vi "Tree.vi"   [LabVIEW 2016, in "Control Experiment SM.lvclass"]
uses:
  Control Experiment SM/Control Experiment SM.lvclass
  <userlib>/LevyLab/Krohn Hite 7008/Instrument.KH7008.lvclass
  <userlib>/LevyLab/Lockin-Multichannel/Instrument.Lockin/Instrument.Lockin.lvclass
  Typedefs/Instrument--enum.ctl
types:
  T1 = typedef "Control Experiment SM.lvclass/Instrument--enum.ctl" = enum16{"----- AFM/EBL -----", "AGILENT", "CYPHER", "Gemini2", "JEOL", "MFP3D", "----- Cryostat -----", "CF900", "DR200", "MNK", "PPMS 1", "PPMS 2", "PPMS 3", "----- Optics -----", "THz 1", "THz 2"}
  T2 = typedef "Control Experiment SM.lvclass/Instruments--cluster.ctl" = cluster{"KH7008":refnum<class "Instrument.KH7008.lvclass">[], "Lockin":refnum<class "Instrument.Lockin.lvclass">, "Temperature":refnum<class "Instrument.Cryostat.lvclass">, "Magnet":refnum<class "Instrument.Cryostat.lvclass">, "Rotator":refnum<class "Instrument.Cryostat.lvclass">, "Level":refnum<class "Instrument.Cryostat.lvclass">, "Capacitance Bridge":refnum<class "Instrument.CBridge.lvclass">, "Optical Delay Line":refnum<class "Instrument.OpticalDelayLine.lvclass">, "Strain Cell":refnum<class "Instrument.Strain.lvclass">, "VNA":refnum<class "Instrument.VNA.lvclass">, "Voltage Source":refnum<class "Instrument.VSource.lvclass">}
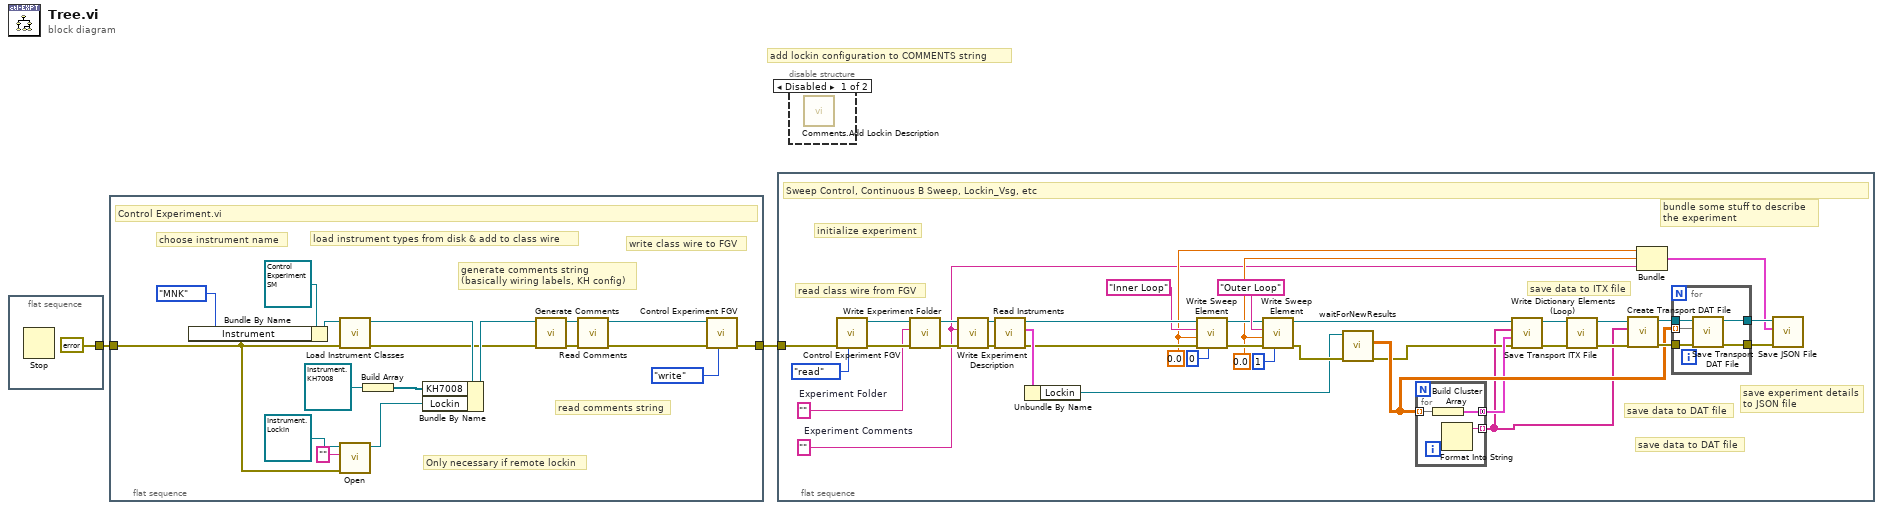
[diagram p0: block diagram]
diagram:
  # "add lockin configuration to COMMENTS string"
  n1 = flat-sequence {
    tunnel: [errorcluster {"status"=FALSE, "code"=0, "source"=""} ("error in (no error)")] -> w2
    frame #0 {
      n2 = Stop() -> ()  [unwired: 1 in]
    }
  }
  n3 = flat-sequence {
    tunnel: w2 -> [w10]
    tunnel: [w9] -> w1
    frame #0 {
      # "choose instrument name"
      # "Only necessary if remote lockin"
      # "write class wire to FGV"
      # "read comments string"
      # "generate comments string\n(basically wiring labels, KH config)"
      # "load instrument types from disk & add to class wire"
      # "Control Experiment.vi"
      n4 = Bundle By Name(cluster=refnum<class "Control Experiment SM.lvclass"> refnum ("Control Experiment.lvclass"), "Instrument"=Instrument--enum."MNK" ("Experiment.Instrument")) -> (w6:refnum<class "Control Experiment SM.lvclass">)
      n5 = call "Load Instrument Classes.vi"("error in (no error)"=w10, "Control Experiment.lvclass"=w6) -> ("error out"=w14:errorcluster, "Control Experiment out"=w16:refnum<class "Control Experiment SM.lvclass">)  [unwired: 8 in]
      n6 = call-dynamic "Open.vi"("error in (no error)"=w10, "Address"="", "Instrument.Lockin in"=refnum<class "Instrument.Lockin.lvclass"> refnum ("Instruments.Lockin")) -> ("Instrument.Lockin out"=w18:refnum<class "Instrument.Lockin.lvclass">)  [unwired: 7 in, 1 out]
      n7 = Build Array(refnum<class "Instrument.KH7008.lvclass"> refnum ("Instruments.KH7008")) -> (w4:refnum<class "Instrument.KH7008.lvclass">[])
      n8 = Bundle By Name(cluster=w16, "KH7008"=w4, "Lockin"=w18) -> (w15:refnum<class "Control Experiment SM.lvclass">)
      n9 = call "Generate Comments.vi"("error in (no error)"=w14, "Control Experiment"=w15) -> ("error out"=w21:errorcluster, "Control Experiment out"=w20:refnum<class "Control Experiment SM.lvclass">)  [unwired: 6 in, 1 out]
      n10 = call "Read Comments.vi"("error in (no error)"=w21, "Control Experiment in"=w20) -> ("error out"=w13:errorcluster, "Control Experiment out"=w12:refnum<class "Control Experiment SM.lvclass">)  [unwired: 7 in, 1 out]
      n11 = call "Control Experiment FGV.vi"("Function"=enum16{"read", "write"}."write", "error in (no error)"=w13, "Control Experiment.lvclass"=w12) -> ("error out"=w9:errorcluster)  [unwired: 7 in, 1 out]
    }
  }
  n12 = flat-sequence {
    tunnel: w1 -> [w58]
    frame #0 {
      w31 = ""  # Experiment Comments
      w30 = ""  # Experiment Folder
      w32 = 0.0
      w33 = 0.0
      # "initialize experiment"
      # "save experiment details\nto JSON file"
      # "save data to DAT file"
      # "save data to DAT file"
      # "save data to ITX file"
      # "bundle some stuff to describe\nthe experiment"
      # "read class wire from FGV"
      # "Sweep Control, Continuous B Sweep, Lockin_Vsg, etc"
      n13 = call "Control Experiment FGV.vi"("Function"=enum16{"read", "write"}."read", "error in (no error)"=w58) -> ("error out"=w54:errorcluster, "Control Experiment.lvclass out"=w53:refnum<class "Control Experiment SM.lvclass">)  [unwired: 8 in]
      n14 = call "Write Experiment Folder.vi"("error in (no error)"=w54, "Experiment Folder"=w30, "Control Experiment in"=w53) -> ("error out"=w55:errorcluster, "Control Experiment out"=w56:refnum<class "Control Experiment SM.lvclass">)  [unwired: 7 in]
      n15 = call "Write Experiment Description.vi"("error in (no error)"=w55, "Experiment Description"=w31, "Control Experiment in"=w56) -> ("error out"=w52:errorcluster, "Control Experiment out"=w51:refnum<class "Control Experiment SM.lvclass">)  [unwired: 7 in]
      n16 = call "Read Instruments.vi"("error in (no error)"=w52, "Control Experiment in"=w51) -> ("error out"=w49:errorcluster, "Instruments"=w50:T2, "Control Experiment out"=w48:refnum<class "Control Experiment SM.lvclass">)  [unwired: 7 in]
      n17 = Unbundle By Name(w50) -> ("Lockin"=w29:refnum<class "Instrument.Lockin.lvclass">)
      n18 = call "Write Sweep Element.vi"("loop index"=0, "error in (no error)"=w49, "value"=w33, "key"="Inner Loop", "Control Experiment in"=w48) -> ("error out"=w42:errorcluster, "Control Experiment out"=w43:refnum<class "Control Experiment SM.lvclass">)  [unwired: 5 in]
      n19 = call "Write Sweep Element.vi"("loop index"=1, "error in (no error)"=w42, "value"=w32, "key"="Outer Loop", "Control Experiment in"=w43) -> ("error out"=w41:errorcluster, "Control Experiment out"=w26:refnum<class "Control Experiment SM.lvclass">)  [unwired: 5 in]
      n20 = call <userlib>:"waitForNewResults.vi"("error in (no error)"=w41, "Instrument.Lockin in"=w29) -> ("error out"=w24:errorcluster, "Results"=w28:dbl[][])  [unwired: 7 in, 1 out]
      n21 = for {
        tunnel: w28 -> [w67] mode=indexing
        tunnel: [w66] -> w27 mode=concatenating
        tunnel: [w64] -> w22 mode=indexing
        i -> [w65]
        n22 = Build Cluster Array(w67) -> (w66:cluster{"Results":dbl[]}[])
        n23 = Format Into String(w65) -> (resulting string=w64:string)  [unwired: 3 in, 1 out]
      }
      n24 = call "Write Dictionary Elements (Loop).vi"("error in (no error)"=w24, "values"=w27, "keys"=w22, "Control Experiment in"=w26) -> ("error out"=w23:errorcluster, "Control Experiment out"=w25:refnum<class "Control Experiment SM.lvclass">)  [unwired: 6 in]
      n25 = call "Save Transport ITX File.vi"("error in (no error)"=w23, "Control Experiment in"=w25) -> ("error out"=w39:errorcluster, "Control Experiment out"=w40:refnum<class "Control Experiment SM.lvclass">)  [unwired: 8 in]
      n26 = call "Create Transport DAT File.vi"("error in (no error)"=w39, "Wavenames"=w22, "Control Experiment in"=w40) -> ("error out"=w37:errorcluster, "Control Experiment out"=w38:refnum<class "Control Experiment SM.lvclass">)  [unwired: 7 in]
      n27 = Bundle(w33, w32, "Experiment Comments"=w31) -> (w34:cluster{dbl, dbl, "Experiment Comments":string})  [unwired: 1 in]
      n28 = for {
        tunnel: w28 -> [w59] mode=indexing
        tunnel: w38 -> [w63]
        tunnel: [w61] -> w36
        tunnel: w37 -> [w62]
        tunnel: [w60] -> w35
        n29 = call "Save Transport DAT File.vi"("error in (no error)"=w62, "Data (Row)"=w59, "Control Experiment in"=w63) -> ("error out"=w60:errorcluster, "Control Experiment out"=w61:refnum<class "Control Experiment SM.lvclass">)  [unwired: 7 in]
      }
      n30 = call "Save JSON File.vi"("error in (no error)"=w35, "Data"=w34, "Control Experiment in"=w36) -> ()  [unwired: 6 in, 3 out]
    }
  }
  n31 = disable-structure shown="Disabled" {
    frame Disabled {
      n32 = call "Comments.Add Lockin Description.vi"() -> ()  [unwired: 9 in, 2 out]
    }
    frame Enabled {
    }
  }
